vi "rotate coordinates about axis from origin.vi"(8 "Angle (CCW)":dbl(knob) scale=0.0..3.14, 10 "Point to rotate":dbl[](array[numeric]), 11 "Rotation axis vector":dbl[](array[numeric])) -> (2 "New position":dbl[](array[numeric]))   [LabVIEW 2018]
doc: "Rotates a point about an axis in 3D space. Axis is defined by the vector between \"Rotation axis vector\" input and the origin."
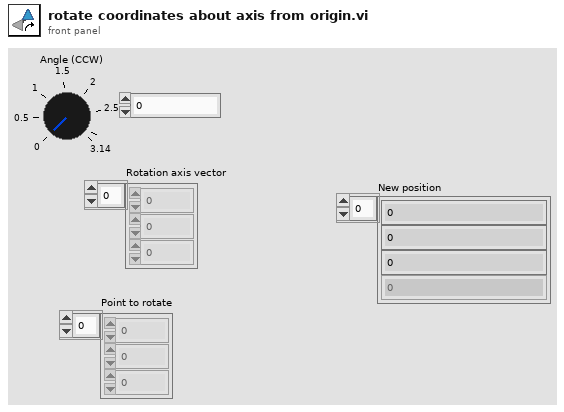
[diagram p1: front panel]
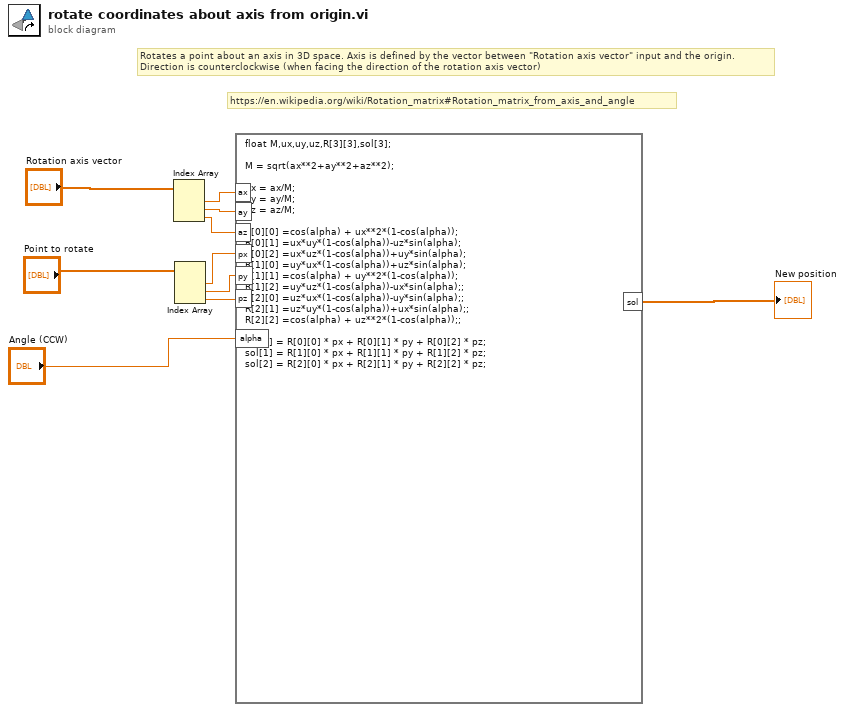
[diagram p0: block diagram]
diagram:
  # "https://en.wikipedia.org/wiki/Rotation_matrix#Rotation_matrix_from_axis_and_angle"
  # "Rotates a point about an axis in 3D space. Axis is defined by the vector between \"Rotation axis vector\" input and the origin.\nDirection is counterclockwise (when facing the direction of the rotation axis vector)"
  n1 = Index Array(array="Rotation axis vector") -> (element #1=w10:dbl, element #2=w9:dbl, element #3=w8:dbl)  [unwired: 3 in]
  n2 = Index Array(array="Point to rotate") -> (element #1=w6:dbl, element #2=w5:dbl, element #3=w4:dbl)  [unwired: 3 in]
  n3 = formula code="float M,ux,uy,uz,R[3][3],sol[3];\n\nM = sqrt(ax**2+ay**2+az**2);\n\nux = ax/M;\nuy = ay/M;\nuz = az/M;\n\nR[0][0] =cos(alpha) + ux**2*(1-cos(alpha));\nR[0][1] =ux*uy*(1-cos(alpha))-uz*sin(alpha);\nR[0][2] =ux*uz*(1-cos(alpha))+uy*sin(alpha);\nR[1][0] =uy*ux*(1-cos(alpha))+uz*sin(alpha);\nR[1][1] =cos(alpha) + uy**2*(1-cos(alpha));\nR[1][2] =uy*uz*(1-cos(alpha))-ux*sin(alpha);;\nR[2][0] =uz*ux*(1-cos(alpha))-uy*sin(alpha);;\nR[2][1] =uz*uy*(1-cos(alpha))+ux*sin(alpha);;\nR[2][2] =cos(alpha) + uz**2*(1-cos(alpha));;\n\nsol[0] = R[0][0] * px + R[0][1] * py + R[0][2] * pz;\nsol[1] = R[1][0] * px + R[1][1] * py + R[1][2] * pz;\nsol[2] = R[2][0] * px + R[2][1] * py + R[2][2] * pz;"("ax"=w10, "ay"=w9, "az"=w8, "px"=w6, "py"=w5, "pz"=w4, "alpha"="Angle (CCW)") -> ("sol"=→"New position":dbl[])
